vi "Ejercicio_05_Maquina de estados.vi"() -> ()   [LabVIEW 2025]
panel:
  in  "stop":bool
  in  "Vaciado":bool
  in  "DL2":bool
  in  "DL1":bool
  in  "SP 3":bool
  in  "SP2":bool
  in  "SP1":bool
  out "V3":bool
  out "M":bool
  out "V1":bool
  out "V2":bool
  out "Vb":bool
  out "Va":bool=TRUE
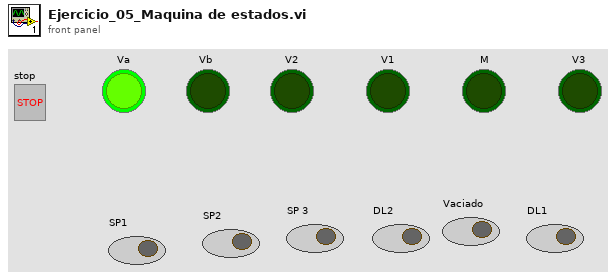
[diagram p1: front panel]
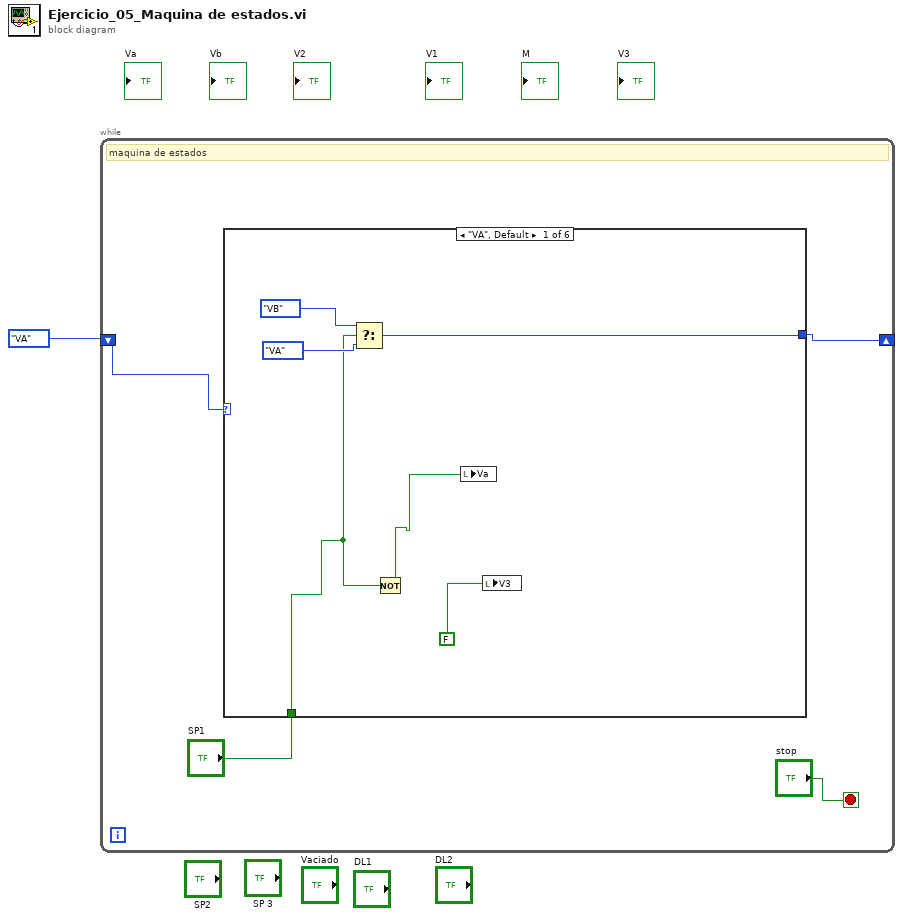
[diagram p0: block diagram]
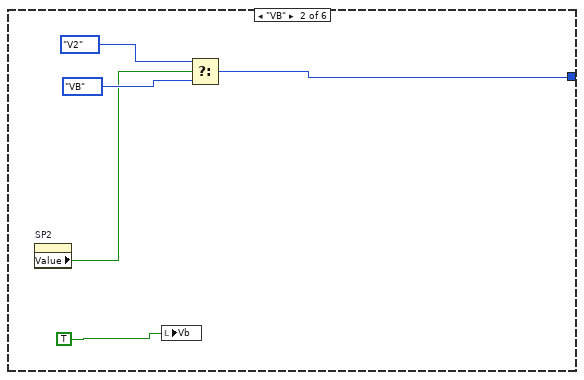
[diagram p2: hidden frame]
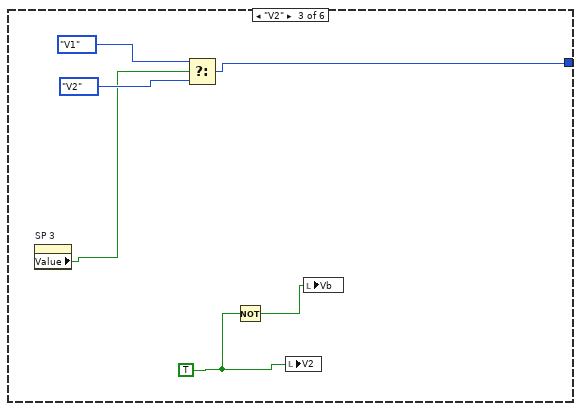
[diagram p3: hidden frame]
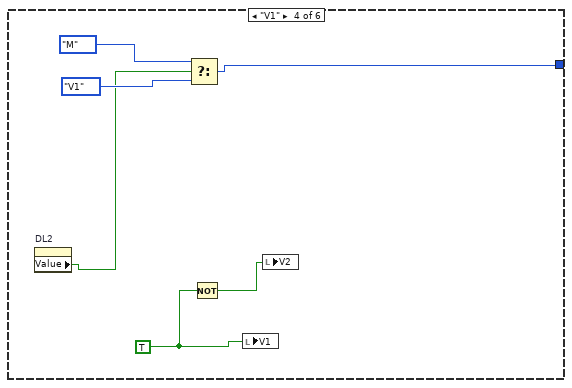
[diagram p4: hidden frame]
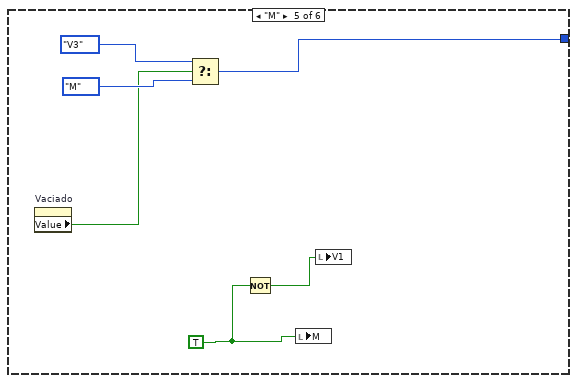
[diagram p5: hidden frame]
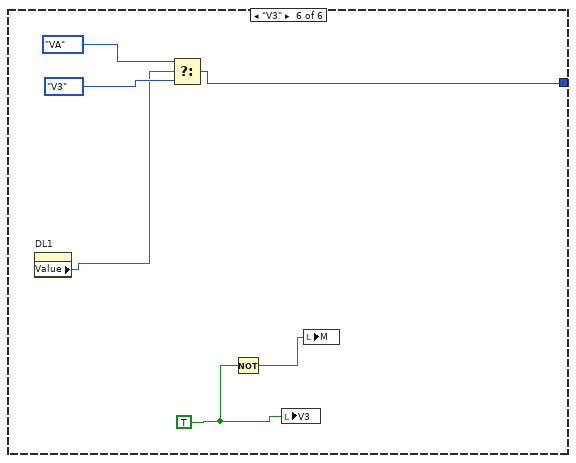
[diagram p6: hidden frame]
diagram:
  n1 = while {
    shift-right: [w4] -> _
    shift-left: enum16{"VA", "VB", "V2", "V1", "M", "V3"}."VA" -> [w5]
    stop <- "stop" stop-if-true
    # "maquina de estados"
    n2 = case shown="\"VA\", Default" w5 {
      tunnel: [w9 w14 w20 w26 w32 w38] -> w4
      tunnel: "SP1" -> [w8 _ _ _ _ _]
      frame "VA", Default {
        n3 = Select(t=enum16{"VA", "VB", "V2", "V1", "M", "V3"}."VB", s=w8, f=enum16{"VA", "VB", "V2", "V1", "M", "V3"}."VA") -> (s? t:f=w9:enum16{"VA", "VB", "V2", "V1", "M", "V3"})
        n4 = Not(x=w8) -> (.not. x?=w7:bool)
        n5 = local write "Va"(w7) -> ()
        n6 = local write "V3"(FALSE) -> ()
      }
      frame "VB" {
        n7 = property on="SP2" class="Bool (strict)"() -> ("Value"=w12:bool)  [unwired: 2 in, 2 out]
        n8 = local write "Vb"(TRUE) -> ()
        n9 = Select(t=enum16{"VA", "VB", "V2", "V1", "M", "V3"}."V2", s=w12, f=enum16{"VA", "VB", "V2", "V1", "M", "V3"}."VB") -> (s? t:f=w14:enum16{"VA", "VB", "V2", "V1", "M", "V3"})
      }
      frame "V2" {
        w18 = TRUE
        n10 = property on="SP 3" class="Bool (strict)"() -> ("Value"=w19:bool)  [unwired: 2 in, 2 out]
        n11 = Select(t=enum16{"VA", "VB", "V2", "V1", "M", "V3"}."V1", s=w19, f=enum16{"VA", "VB", "V2", "V1", "M", "V3"}."V2") -> (s? t:f=w20:enum16{"VA", "VB", "V2", "V1", "M", "V3"})
        n12 = Not(x=w18) -> (.not. x?=w17:bool)
        n13 = local write "V2"(w18) -> ()
        n14 = local write "Vb"(w17) -> ()
      }
      frame "V1" {
        w23 = TRUE
        n15 = property on="DL2" class="Bool (strict)"() -> ("Value"=w25:bool)  [unwired: 2 in, 2 out]
        n16 = Select(t=enum16{"VA", "VB", "V2", "V1", "M", "V3"}."M", s=w25, f=enum16{"VA", "VB", "V2", "V1", "M", "V3"}."V1") -> (s? t:f=w26:enum16{"VA", "VB", "V2", "V1", "M", "V3"})
        n17 = Not(x=w23) -> (.not. x?=w24:bool)
        n18 = local write "V1"(w23) -> ()
        n19 = local write "V2"(w24) -> ()
      }
      frame "M" {
        w30 = TRUE
        n20 = property on="Vaciado" class="Bool (strict)"() -> ("Value"=w31:bool)  [unwired: 2 in, 2 out]
        n21 = Select(t=enum16{"VA", "VB", "V2", "V1", "M", "V3"}."V3", s=w31, f=enum16{"VA", "VB", "V2", "V1", "M", "V3"}."M") -> (s? t:f=w32:enum16{"VA", "VB", "V2", "V1", "M", "V3"})
        n22 = Not(x=w30) -> (.not. x?=w29:bool)
        n23 = local write "M"(w30) -> ()
        n24 = local write "V1"(w29) -> ()
      }
      frame "V3" {
        w36 = TRUE
        n25 = property on="DL1" class="Bool (strict)"() -> ("Value"=w37:bool)  [unwired: 2 in, 2 out]
        n26 = Select(t=enum16{"VA", "VB", "V2", "V1", "M", "V3"}."VA", s=w37, f=enum16{"VA", "VB", "V2", "V1", "M", "V3"}."V3") -> (s? t:f=w38:enum16{"VA", "VB", "V2", "V1", "M", "V3"})
        n27 = Not(x=w36) -> (.not. x?=w35:bool)
        n28 = local write "V3"(w36) -> ()
        n29 = local write "M"(w35) -> ()
      }
    }
  }
